vi "Get Project Data.vi"(8 "error in":errorcluster, 10 "Target Selection":string, 11 "Project Selection":string) -> (0 "error out":errorcluster, 3 "Project Data":T1)   [LabVIEW 2020, in "ConstantErrorsMaker.lvlib"]
uses:
  ConstantErrorsMaker.lvlib
  Project Data--cluster.ctl
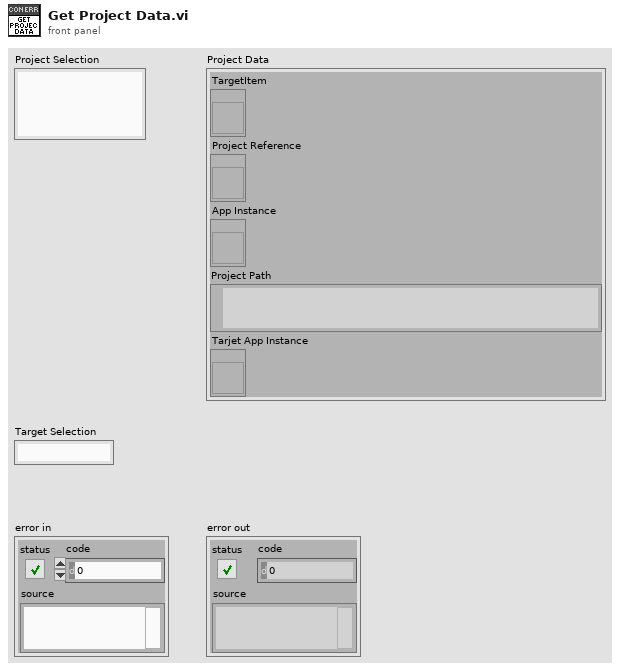
[diagram p1: front panel]
types:
  T1 = typedef "ConstantErrorsMaker.lvlib/Project Data--cluster.ctl" = cluster{"TargetItem":refnum<vi>, "Project Reference":refnum<vi>, "App Instance":refnum<vi>, "Project Path":path, "Tarjet App Instance":refnum<vi>}
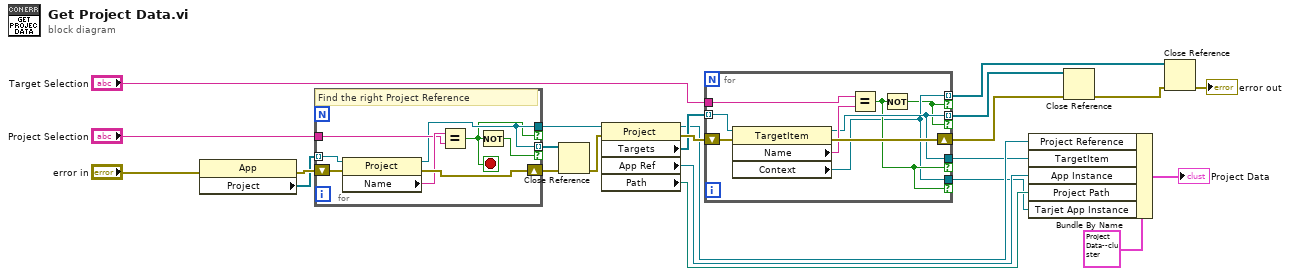
[diagram p0: block diagram]
diagram:
  n1 = property class="App"(error in="error in") -> (error out=w21:errorcluster, "Project"=w14:refnum<vi>[])  [unwired: 1 in, 1 out]
  n2 = for {
    tunnel: [w27] -> w9 if=w26
    tunnel: "Project Selection" -> [w28]
    tunnel: [w27] -> w13 mode=indexing if=w25
    tunnel: w14 -> [w24] mode=indexing
    shift-right: [w31] -> w22
    shift-left: w21 -> [w30]
    stop <- w26 stop-if-true
    # "Find the right Project Reference"
    n3 = property class="Project"(reference=w24, error in=w30) -> (reference out=w27:refnum<vi>, error out=w31:errorcluster, "Name"=w29:string)
    n4 = Equal?(x=w29, y=w28) -> (x = y?=w26:bool)
    n5 = Not(x=w26) -> (.not. x?=w25:bool)
  }
  n6 = Close Reference(reference=w13, error in (no error)=w22) -> (error out=w17:errorcluster)
  n7 = property class="Project"(reference=w9, error in=w17) -> (reference out=w6:refnum<vi>, error out=w19:errorcluster, "Targets"=w11:refnum<vi>[], "App Ref"=w4:refnum<vi>, "Path"=w3:path)
  n8 = for {
    tunnel: w11 -> [w38] mode=indexing
    tunnel: [w36] -> w5 if=w35
    tunnel: [w36] -> w12 mode=indexing if=w33
    shift-right: [w39] -> w18
    shift-left: w19 -> [w40]
    tunnel: [w34] -> w1 if=w35
    tunnel: [w34] -> w10 mode=indexing if=w33
    tunnel: "Target Selection" -> [w32]
    n9 = property class="TargetItem"(reference=w38, error in=w40) -> (reference out=w36:refnum<vi>, error out=w39:errorcluster, "Name"=w37:string, "Context"=w34:refnum<vi>)
    n10 = Equal?(x=w32, y=w37) -> (x = y?=w35:bool)
    n11 = Not(x=w35) -> (.not. x?=w33:bool)
  }
  n12 = Bundle By Name(cluster=T1 {"TargetItem"=refnum, "Project Reference"=refnum, "App Instance"=refnum, "Project Path"=path "", "Tarjet App Instance"=refnum} ("Project Data"), "Project Reference"=w6, "TargetItem"=w5, "App Instance"=w4, "Project Path"=w3, "Tarjet App Instance"=w1) -> (→"Project Data":T1)
  n13 = Close Reference(reference=w12, error in (no error)=w18) -> (error out=w20:errorcluster)
  n14 = Close Reference(reference=w10, error in (no error)=w20) -> (error out=→"error out":errorcluster)
